vi "WriteSweep.vi"(6 "unit":string, 7 "sweep valid":bool, 8 "error in (no error)":errorcluster, 9 "sweep":cluster{"frequency":dbl, "amplitude":dbl}[](array[cluster]), 10 "channel":string, 11 "map":T1) -> (0 "error out":errorcluster, 3 "map out":T1)   [LabVIEW 2017, in "EmsaAcquisition.lvlib"]
uses:
  <vilib>/addons/InsightCM/Devices/Shared/Emsa/EmsaAcquisition/EmsaAcquisition.lvlib
  <vilib>/addons/PointValueMap/controls/PointMap.ctl
  <vilib>/addons/PointValueMap/subVIs/Point_Write_string.vi
  <vilib>/addons/PointValueMap/PointValueMap.lvlib
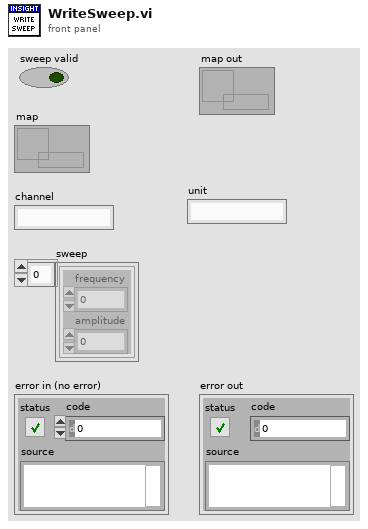
[diagram p1: front panel]
types:
  T1 = typedef "PointValueMap.lvlib/PointMap.ctl" = refnum<data-value>
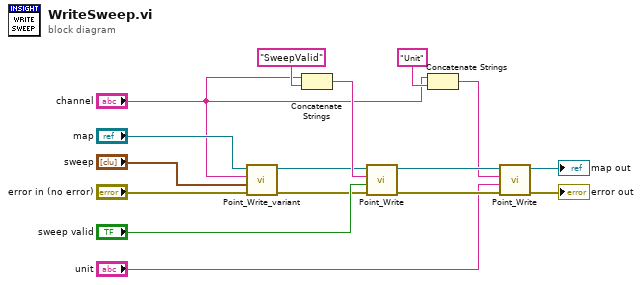
[diagram p0: block diagram]
diagram:
  n1 = call <vilib>:"Point_Write_variant.vi"("Error In"="error in (no error)", "Value"="sweep", "Tag"="channel", "Map"="map") -> ("Error Out"=w13:errorcluster, "Map Out"=w12:T1)  [unwired: 6 in]
  n2 = Concatenate Strings("channel", "SweepValid" ("Tag")) -> (w15:string)
  n3 = call-poly <vilib>:"Point_Write.vi"("Error In"=w13, "Value"="sweep valid", "Tag"=w15, "Map"=w12) -> ("Error Out"=w8:errorcluster, "Map Out"=w6:T1)  [unwired: 6 in]
  n4 = Concatenate Strings("channel", "Unit" ("Tag")) -> (w2:string)
  n5 = call-poly <vilib>:"Point_Write.vi"("Error In"=w8, "Value"="unit", "Tag"=w2, "Map"=w6) -> ("Error Out"=→"error out":errorcluster, "Map Out"=→"map out":T1)  [unwired: 6 in]
